vi "Range to mA GS Span.vi"(5 "Range and span":T1={"GS Range (0 : 4-20mA)"=0, "Enable Span (False)"=FALSE, "Lower Span (4.000)"=4.0, "Upper Span (20.000)"=20.0, "Bias (0)"=0.0} {"Upper Span (20.000)" min=-99999.0 max=99999.0 step=1.0 format="%.3g"; "Lower Span (4.000)" min=-99999.0 max=99999.0 step=1.0 format="%.3g"; "GS Range (0 : 4-20mA)" items=["4-20mA"]}, 9 "Floating Point Position (2)":i32 min=0 max=5) -> (6 "Lower Span":i32=-2000 min=-99999 max=99999 step=1, 8 "Upper Span":i32=2000 min=-99999 max=99999 step=1, 10 "Bias":i32)   [LabVIEW 2020, in "Yokogawa GX Series.lvlib"]
doc: "This VI gets the GS span value from the range."
uses:
  <instrlib>/Yokogawa GX Series/Yokogawa GX Series.lvlib
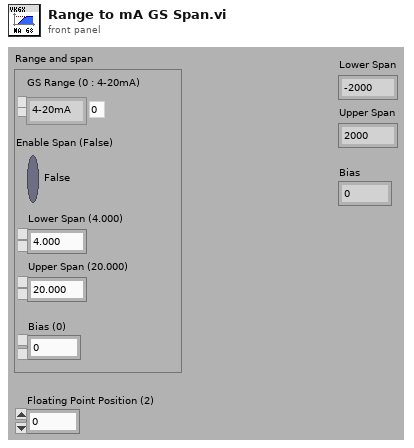
[diagram p1: front panel]
types:
  T1 = cluster{"GS Range (0 : 4-20mA)":i32, "Enable Span (False)":bool, "Lower Span (4.000)":dbl, "Upper Span (20.000)":dbl, "Bias (0)":dbl}
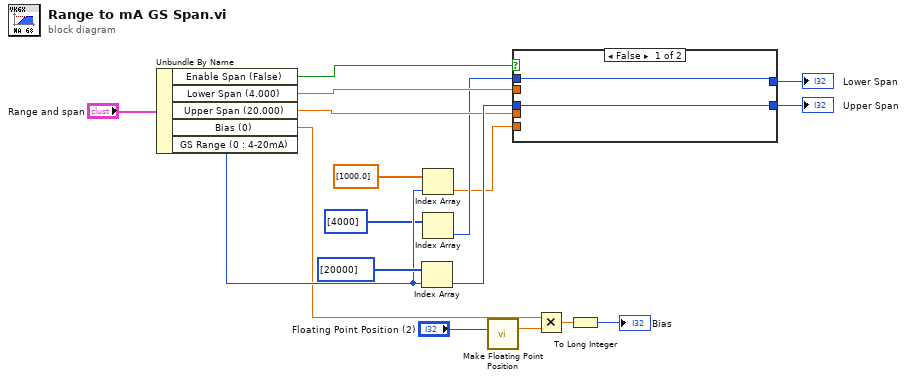
[diagram p0: block diagram]
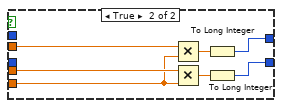
[diagram p2: hidden frame]
diagram:
  n1 = Unbundle By Name("Range and span") -> ("Enable Span (False)"=w10:bool, "Lower Span (4.000)"=w11:dbl, "Upper Span (20.000)"=w12:dbl, "Bias (0)"=w1:dbl, "GS Range (0 : 4-20mA)"=w9:i32)
  n2 = Index Array(array=i32[] [20000], index=w9) -> (element=w18:i32)
  n3 = Index Array(array=dbl[] [1000.0], index=w9) -> (element=w6:dbl)
  n4 = Index Array(array=i32[] [4000]) -> (element=w7:i32)  [unwired: 1 in]
  n5 = call <instrlib>:"Make Floating Point Position.vi"("Floating Point Position (2)"="Floating Point Position (2)") -> ("Times"=w4:dbl)  [unwired: 14 in]
  n6 = case shown="False" w10 {
    tunnel: w11 -> [_ w26]
    tunnel: w12 -> [_ w25]
    tunnel: [w19 w23] -> w17
    tunnel: [w20 w22] -> w16
    tunnel: w18 -> [w20 _]
    tunnel: w6 -> [_ w21]
    tunnel: w7 -> [w19 _]
    frame False {
    }
    frame True {
      n7 = Multiply(x=w26, y=w21) -> (x*y=w27:dbl)
      n8 = Multiply(x=w25, y=w21) -> (x*y=w24:dbl)
      n9 = To Long Integer(number=w27) -> (32bit integer=w23:i32)
      n10 = To Long Integer(number=w24) -> (32bit integer=w22:i32)
    }
  }
  "Lower Span" <- w17
  "Upper Span" <- w16
  n11 = Multiply(x=w1, y=w4) -> (x*y=w3:dbl)
  n12 = To Long Integer(number=w3) -> (32bit integer=→"Bias":i32)
